vi "Speech recognition.vi"() -> ()   [LabVIEW 2018]
panel:
  out "Recognizing...":bool
  out "Recording...":bool
  out "Waveform Graph":dynamicdata(graph)
  out "return value":string
  in  "temp path":path=path "D:/test.wav"
  # "LabVIEW  - Google Speech Recognition API (Python)"
  # "This is a path to a temp wav file that is stored by labview.  \nI couldn't figure out how to pass arrays directly into Python, so this is a workaround."
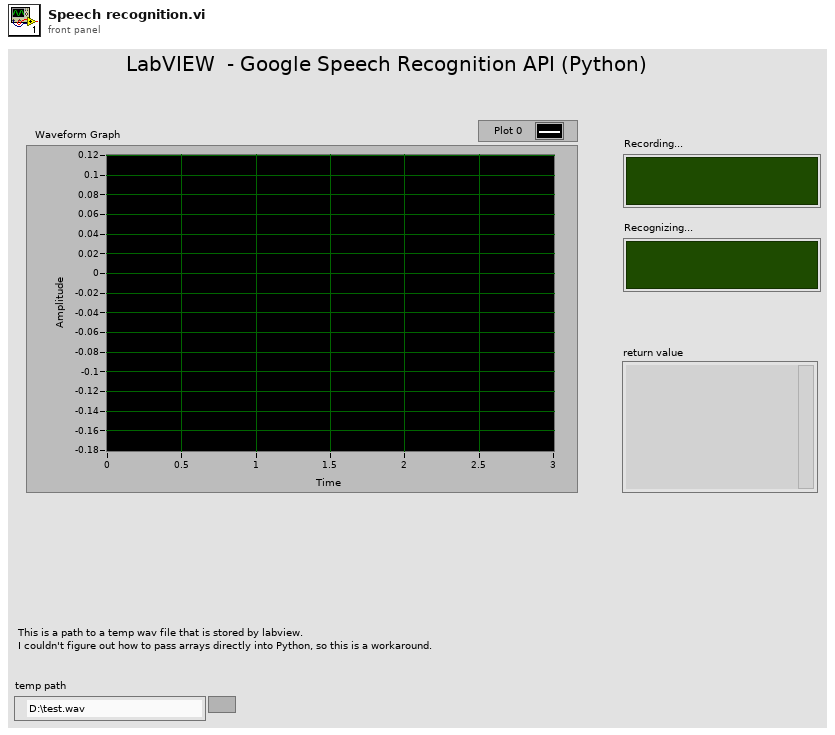
[diagram p1: front panel]
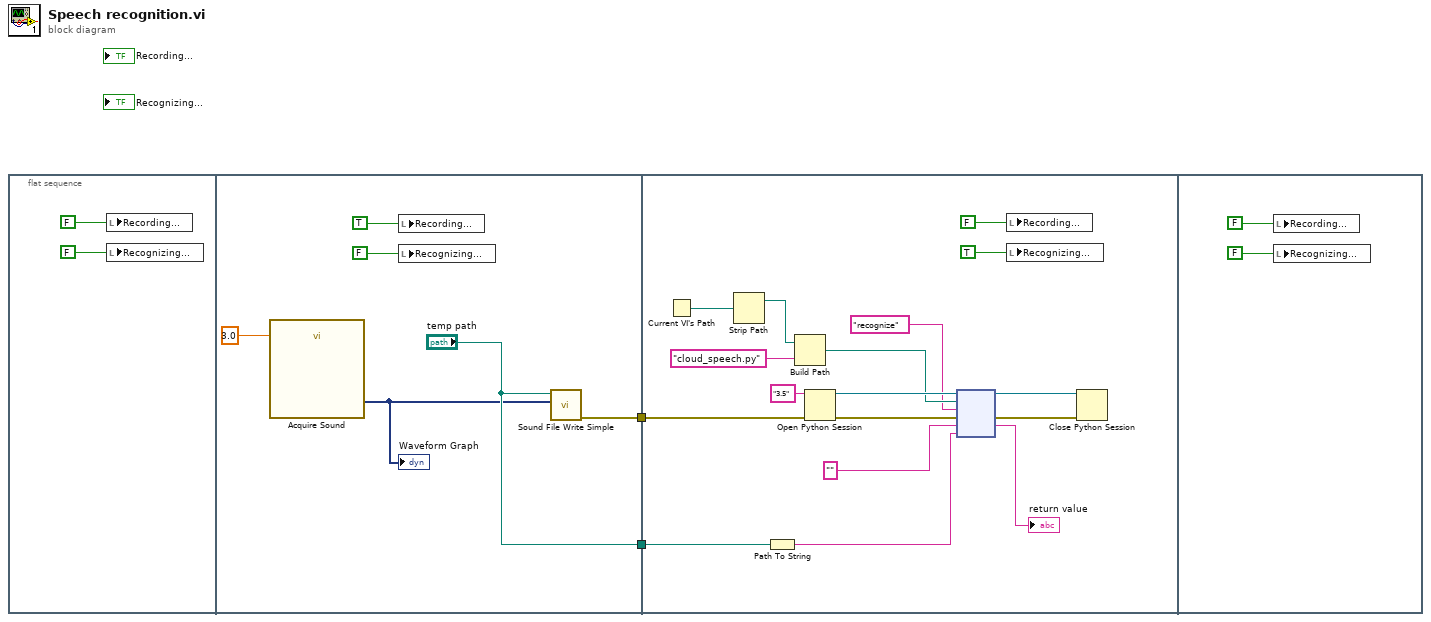
[diagram p0: block diagram]
diagram:
  n1 = flat-sequence {
    tunnel: [w10] -> w2
    tunnel: ["temp path"] -> w1
    tunnel: w2 -> [w17]
    tunnel: w1 -> [w13]
    frame #0 {
      n2 = local write "Recording..."(FALSE ("Recording...")) -> ()
      n3 = local write "Recognizing..."(FALSE ("Recognizing...")) -> ()
    }
    frame #1 {
      n4 = call "Acquire Sound"("Duration (s)"=3.0) -> ("Data"=w7:dynamicdata)  [unwired: 17 in, 1 out]
      "Waveform Graph" <- w7
      n5 = local write "Recording..."(TRUE ("Recording...")) -> ()
      n6 = local write "Recognizing..."(FALSE ("Recognizing...")) -> ()
      n7 = call <vilib>:"Sound File Write Simple.vi"("data"=w7, "path"="temp path") -> ("error out"=w10:errorcluster)  [unwired: 8 in, 1 out]
    }
    frame #2 {
      n8 = Current VI's Path() -> (path=w27:path)
      n9 = Strip Path(path=w27) -> (stripped path=w18:path)  [unwired: 1 out]
      n10 = Path To String(path=w13) -> (string=w14:string)
      n11 = Build Path(base path=w18, name or relative path="cloud_speech.py") -> (appended path=w22:path)
      n12 = Open Python Session(python version="3.5" ("Python version"), 3:w17) -> (session out=w24:refnum<k35>, error out=w16:errorcluster)  [unwired: 1 in]
      n13 = node(w24, w22, "recognize" ("function name"), w16, "" ("Python version"), w14) -> (w23:refnum<k35>, w15:errorcluster, →"return value":string)  [unwired: 1 in, 2 out]
      n14 = local write "Recording..."(FALSE ("Recording...")) -> ()
      n15 = local write "Recognizing..."(TRUE ("Recognizing...")) -> ()
      n16 = Close Python Session(session in=w23, error in=w15) -> ()  [unwired: 1 out]
    }
    frame #3 {
      n17 = local write "Recording..."(FALSE ("Recording...")) -> ()
      n18 = local write "Recognizing..."(FALSE ("Recognizing...")) -> ()
    }
  }
